vi "CalibrateMicroscopeGUI.vi"() -> ()   [LabVIEW 2011]
panel:
  in  "cam y-pixel center":dbl=740.0
  in  "cam x-pixel center":dbl=252.0
  out "cam.calibration.basis":string="0,-0.0014617169,0,0.0042923434;1280,0.005962877,0,0.0042923434;0,-0.0014617169,1024,-0.0016473318"
  in  "move[m]":dbl=0.0002
  in  "cam position2[Pixel]":dbl=258.0
  in  "cam position1[pixel]":dbl=1120.0
  in  "Objektiv":dbl=25.0
  out "Pixelsize [m]":dbl=5.80046403712297e-06
  out "mmII/s^2":dbl=368613.53802120243
  out "°opt/s^2":dbl=640000000.0
  out "Estimate m/bit":dbl=7.030745277809189e-07
  in  "6210 Galvo +-°mech":dbl=20.0
  out "galvo.orientation":string="0,0.0007778175,0,0.0006363961;1,0.7078845986,0,0.7077431773;0,0.7078845986,1,-0.7064703851"
  in  "Galvo.orientation (Center first)":T1={"Center"={-0.001, -0.0001}, "Rotate (grad)"=-45.0, "MirrorY"=TRUE, "Scale"=1.0}
  in  "Max A":dbl=5.0
  in  "cam y-pixels":dbl=1024.0
  in  "cam x-pixels":dbl=1280.0
  in  "6210 Galvo °mech/s^2/A":dbl=64000000.0
  in  "f Scanlens [mm]":dbl=33.0
  # "galvo.maxacceleration"
  # "do cam image, get feature, move stage, find pixel of feature again"
  # "find center (scan and find feature), do camera image, find feature again get pixels"
  # "copy to Variable, change, reastart cam driver, make image load into definescan"
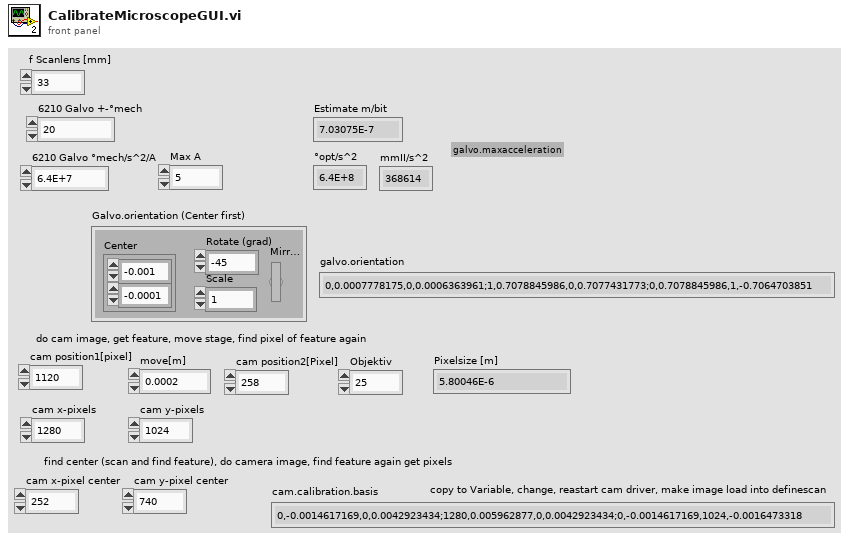
[diagram p1: front panel]
types:
  T1 = cluster{"Center":cluster{dbl, dbl}, "Rotate (grad)":dbl, "MirrorY":bool, "Scale":dbl}
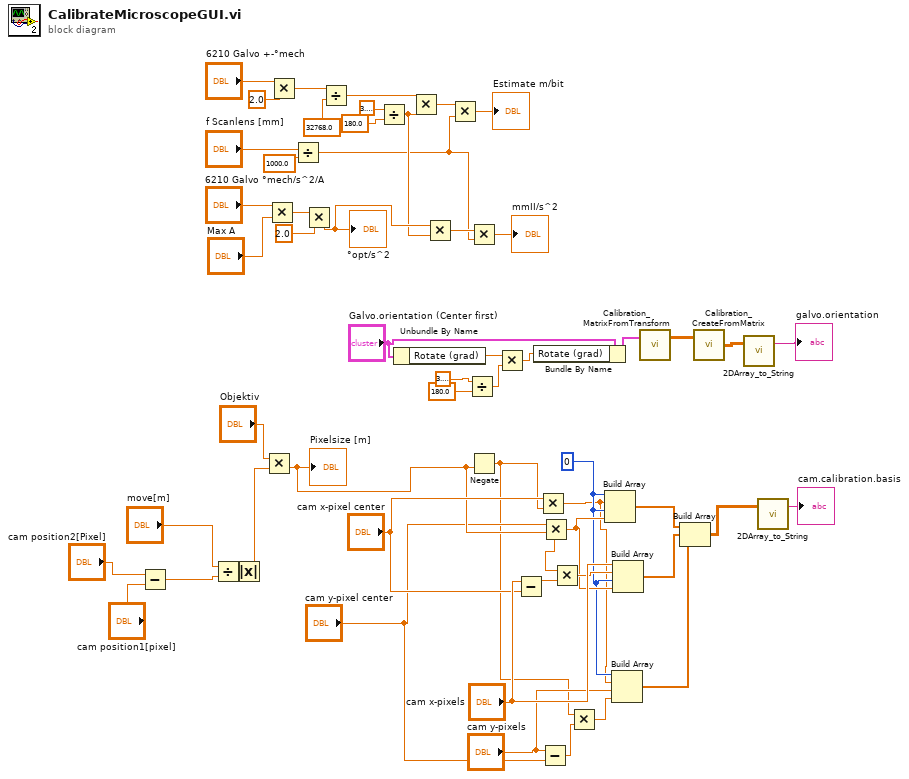
[diagram p0: block diagram]
diagram:
  w6 = 0
  n1 = Subtract(x="cam position2[Pixel]", y="cam position1[pixel]") -> (x-y=w23:dbl)
  n2 = Divide(x="move[m]", y=w23) -> (x/y=w21:dbl)
  n3 = Absolute Value(x=w21) -> (abs(x)=w19:dbl)
  n4 = Multiply(x="Objektiv", y=w19) -> (x*y=w14:dbl)
  "Pixelsize [m]" <- w14
  n5 = Multiply(x="6210 Galvo °mech/s^2/A", y="Max A") -> (x*y=w32:dbl)
  n6 = Multiply(x="6210 Galvo +-°mech", y=2.0) -> (x*y=w43:dbl)
  n7 = Divide(x="f Scanlens [mm]", y=1000.0) -> (x/y=w27:dbl)
  n8 = Multiply(x=w32, y=2.0) -> (x*y=w30:dbl)
  "°opt/s^2" <- w30
  n9 = Divide(x=w43, y=32768.0) -> (x/y=w39:dbl)
  n10 = Divide(x=3.141592653589793, y=180.0 ("x")) -> (x/y=w29:dbl)
  n11 = Unbundle By Name("Galvo.orientation (Center first)") -> ("Rotate (grad)"=w51:dbl)
  n12 = Multiply(x=w39, y=w29) -> (x*y=w36:dbl)
  n13 = Multiply(x=w30, y=w29) -> (x*y=w28:dbl)
  n14 = Multiply(x=w36, y=w27) -> (x*y=→"Estimate m/bit":dbl)
  n15 = Divide(x=3.141592653589793, y=180.0) -> (x/y=w50:dbl)
  n16 = Multiply(x=w28, y=w27) -> (x*y=→"mmII/s^2":dbl)
  n17 = Negate(x=w14) -> (-x=w2:dbl)
  n18 = Multiply(x=w51, y=w50) -> (x*y=w49:dbl)
  n19 = Subtract(x="cam x-pixels", y="cam x-pixel center") -> (x-y=w15:dbl)
  n20 = Bundle By Name(cluster="Galvo.orientation (Center first)", "Rotate (grad)"=w49) -> (w54:T1)
  n21 = Multiply(x="cam x-pixel center", y=w2) -> (x*y=w5:dbl)
  n22 = Subtract(x="cam y-pixels", y="cam y-pixel center") -> (x-y=w11:dbl)
  n23 = Multiply(x="cam y-pixel center", y=w14) -> (x*y=w10:dbl)
  n24 = Multiply(x=w14, y=w15) -> (x*y=w13:dbl)
  n25 = Multiply(x=w2, y=w11) -> (x*y=w3:dbl)
  n26 = Build Array(w6, w5, w6, w10) -> (w9:dbl[])
  n27 = Build Array(w6, w5, "cam y-pixels", w3) -> (w7:dbl[])
  n28 = Build Array("cam x-pixels", w13, w6, w10) -> (w8:dbl[])
  n29 = call "Calibration_MatrixFromTransform.vi"("Transform (Center first)"=w54) -> ("Linear conversion Matrix"=w48:dbl[][])  [unwired: 2 in]
  n30 = Build Array(w9, w8, w7) -> (w1:dbl[][])
  n31 = call "Calibration_CreateFromMatrix.vi"("Linear conversion Matrix"=w48) -> ("CalibrationCoordinates: x,x',y,y'..."=w46:dbl[][])  [unwired: 1 in]
  n32 = call "2DArray_to_String.vi"("Array"=w46) -> ("String 1"=→"galvo.orientation":string)  [unwired: 3 in, 1 out]
  n33 = call "2DArray_to_String.vi"("Array"=w1) -> ("String 1"=→"cam.calibration.basis":string)  [unwired: 3 in, 1 out]
